vi "function3.vi"   [LabVIEW 2016, in "Test.lvrbt"]
uses:
  Test.lvrbt
  <vilib>/NXT/Block Support/NXT_InputPort.ctl
  <vilib>/NXT/Subs/ColorSensorColors.ctl
  <vilib>/NXT/Hardware/Plugins/Tetrix DC Motor/TetrixDCMotorAddress.ctl
  <vilib>/NXT/Hardware/Plugins/Tetrix 180 deg Servo/Tetrix180ServoAddress.ctl
  <vilib>/NXT/NXTIO Xnodes/NXTIONodeSubVIs/TETRIX IO Move DC Motors.vi
  <vilib>/NXT/Dual Mode Library/Waits/Wait_EV3_Color_Color.vi
  <vilib>/NXT/NXTIO Xnodes/NXTIONodeSubVIs/TETRIX IO Stop DC Motors.vi
  <vilib>/NXT/Dual Mode Library/Waits/Wait_Num.vi
  <vilib>/NXT/Dual Mode Library/Waits/Wait_EV3_Ultrasonic_Centimeter_Closer.vi
  <vilib>/NXT/NXTIO Xnodes/NXTIONodeSubVIs/TETRIX IO Move Servos.vi
  <vilib>/NXT/Subs/LVHSConnector.ctl
  <vilib>/NXT/NXTIO Xnodes/AddressXNode/NXTIOAddress.xnode
  <vilib>/NXT/NXTIO Xnodes/NXTIOXNode/NXTIO.xnode
  <vilib>/NXT/LegoClasses/BrickReference/BrickReference.lvclass
types:
  T1 = typedef "NXT_InputPort.ctl" = u32
  T2 = typedef "ColorSensorColors.ctl" = enum16{"No Color", "Black", "Blue", "Green", "Yellow", "Red", "White", "Brown"}
  T3 = typedef "TetrixDCMotorAddress.ctl" = i32
  T4 = typedef "LVHSConnector.ctl" = refnum<class "BrickReference.lvclass">
  T5 = typedef "Tetrix180ServoAddress.ctl" = i32
  T6 = cluster{"Tetrix180Servo":T5, "Tetrix180Servo":T5, "Tetrix180Servo":T5, "Tetrix180Servo":T5, "Tetrix180Servo":T5}
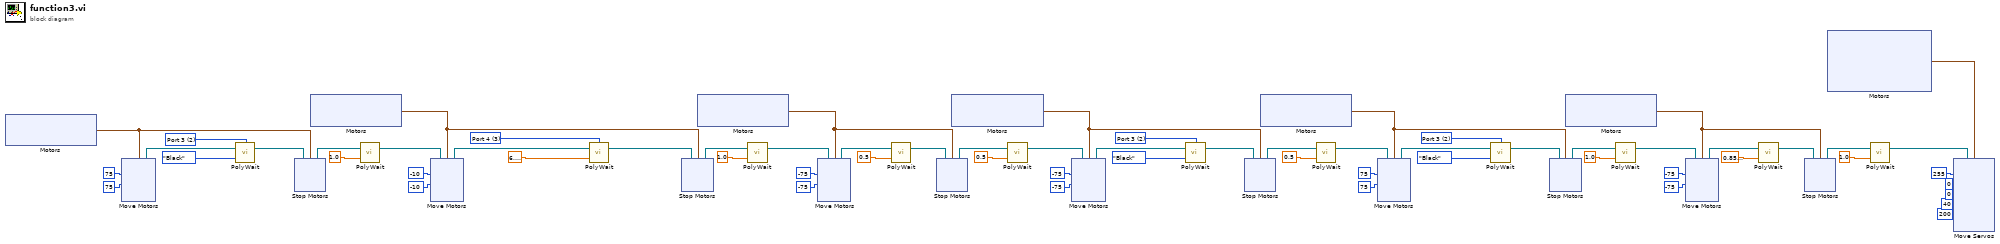
[diagram p0: block diagram]
diagram:
  w25 = T1 2 items=["Port 1", "Port 2", "Port 3", "Port 4"] ("Port (Port 1)")
  w42 = T1 2 items=["Port 1", "Port 2", "Port 3", "Port 4"] ("Port (Port 1)")
  w50 = T1 3 items=["Port 1", "Port 2", "Port 3", "Port 4"] ("Port (Port 1)")
  w60 = T1 2 items=["Port 1", "Port 2", "Port 3", "Port 4"] ("Port (Port 1)")
  n1 = xnode "Motors"() -> ("Motor"=w58:cluster{"TetrixDCMotor":T3, "TetrixDCMotor":T3})
  n2 = xnode "Move Motors"("Power/Speed 2"=i8 75, "Power/Speed 1"=i8 75, "Motors"=w58) -> ("NXT/EV3"=w62:T4)  [unwired: 1 in]
  n3 = call-poly <vilib>:"PolyWait.vi"("Color (Red)"=ColorSensorColors."Black", "NXT/EV3"=w62, "Port (Port 1)"=w60) -> ("NXT/EV3"=w59:T4)  [unwired: 1 in]
  n4 = xnode "Stop Motors"("Motors"=w58, "NXT/EV3"=w59) -> ("NXT/EV3"=w55:T4)
  n5 = xnode "Motors"() -> ("Motor"=w48:cluster{"TetrixDCMotor":T3, "TetrixDCMotor":T3})
  n6 = call-poly <vilib>:"PolyWait.vi"("Time (1 sec)"=sgl 1.0, "NXT/EV3"=w55) -> ("NXT/EV3"=w53:T4)  [unwired: 2 in]
  n7 = xnode "Move Motors"("Power/Speed 2"=i8 -10, "Power/Speed 1"=i8 -10, "Motors"=w48, "NXT/EV3"=w53) -> ("NXT/EV3"=w51:T4)
  n8 = call-poly <vilib>:"PolyWait.vi"("Centimeters (40)"=sgl 6.9 ("Time (1 sec)"), "NXT/EV3"=w51, "Port (Port 1)"=w50) -> ("NXT/EV3"=w49:T4)  [unwired: 1 in]
  n9 = xnode "Stop Motors"("Motors"=w48, "NXT/EV3"=w49) -> ("NXT/EV3"=w46:T4)
  n10 = xnode "Motors"() -> ("Motor"=w34:cluster{"TetrixDCMotor":T3, "TetrixDCMotor":T3})
  n11 = call-poly <vilib>:"PolyWait.vi"("Time (1 sec)"=sgl 1.0, "NXT/EV3"=w46) -> ("NXT/EV3"=w33:T4)  [unwired: 2 in]
  n12 = xnode "Move Motors"("Power/Speed 2"=i8 -75, "Power/Speed 1"=i8 -75, "Motors"=w34, "NXT/EV3"=w33) -> ("NXT/EV3"=w35:T4)
  n13 = call-poly <vilib>:"PolyWait.vi"("Time (1 sec)"=sgl 0.5, "NXT/EV3"=w35) -> ("NXT/EV3"=w36:T4)  [unwired: 2 in]
  n14 = xnode "Stop Motors"("Motors"=w34, "NXT/EV3"=w36) -> ("NXT/EV3"=w30:T4)
  n15 = xnode "Motors"() -> ("Motor"=w39:cluster{"TetrixDCMotor":T3, "TetrixDCMotor":T3})
  n16 = call-poly <vilib>:"PolyWait.vi"("Time (1 sec)"=sgl 0.5, "NXT/EV3"=w30) -> ("NXT/EV3"=w29:T4)  [unwired: 2 in]
  n17 = xnode "Move Motors"("Power/Speed 2"=i8 -75, "Power/Speed 1"=i8 -75, "Motors"=w39, "NXT/EV3"=w29) -> ("NXT/EV3"=w40:T4)
  n18 = call-poly <vilib>:"PolyWait.vi"("Color (Red)"=ColorSensorColors."Black", "NXT/EV3"=w40, "Port (Port 1)"=w42) -> ("NXT/EV3"=w41:T4)  [unwired: 1 in]
  n19 = xnode "Stop Motors"("Motors"=w39, "NXT/EV3"=w41) -> ("NXT/EV3"=w5:T4)
  n20 = xnode "Motors"() -> ("Motor"=w22:cluster{"TetrixDCMotor":T3, "TetrixDCMotor":T3})
  n21 = call-poly <vilib>:"PolyWait.vi"("Time (1 sec)"=sgl 0.5, "NXT/EV3"=w5) -> ("NXT/EV3"=w11:T4)  [unwired: 2 in]
  n22 = xnode "Move Motors"("Power/Speed 2"=i8 75, "Power/Speed 1"=i8 75, "Motors"=w22, "NXT/EV3"=w11) -> ("NXT/EV3"=w23:T4)
  n23 = call-poly <vilib>:"PolyWait.vi"("Color (Red)"=ColorSensorColors."Black", "NXT/EV3"=w23, "Port (Port 1)"=w25) -> ("NXT/EV3"=w24:T4)  [unwired: 1 in]
  n24 = xnode "Stop Motors"("Motors"=w22, "NXT/EV3"=w24) -> ("NXT/EV3"=w20:T4)
  n25 = xnode "Motors"() -> ("Motor"=w13:cluster{"TetrixDCMotor":T3, "TetrixDCMotor":T3})
  n26 = call-poly <vilib>:"PolyWait.vi"("Time (1 sec)"=sgl 1.0, "NXT/EV3"=w20) -> ("NXT/EV3"=w17:T4)  [unwired: 2 in]
  n27 = xnode "Move Motors"("Power/Speed 2"=i8 -75, "Power/Speed 1"=i8 -75, "Motors"=w13, "NXT/EV3"=w17) -> ("NXT/EV3"=w15:T4)
  n28 = call-poly <vilib>:"PolyWait.vi"("Time (1 sec)"=sgl 0.85, "NXT/EV3"=w15) -> ("NXT/EV3"=w14:T4)  [unwired: 2 in]
  n29 = xnode "Stop Motors"("Motors"=w13, "NXT/EV3"=w14) -> ("NXT/EV3"=w10:T4)
  n30 = xnode "Motors"() -> ("Motor"=w7:T6)
  n31 = call-poly <vilib>:"PolyWait.vi"("Time (1 sec)"=sgl 1.0, "NXT/EV3"=w10) -> ("NXT/EV3"=w8:T4)  [unwired: 2 in]
  n32 = xnode "Move Servos"("Position 5"=u8 200, "Position 4"=u8 40, "Position 3"=u8 0, "Position 2"=u8 0, "Position 1"=u8 255, "Motors"=w7, "NXT/EV3"=w8) -> ()  [unwired: 1 out]
